vi "Set Control Visibility.vi"(9 "Visible":bool, 10 "index":i32, 11 "Waveform":refnum<vi>) -> ()   [LabVIEW 2016, in "M1M3SupportEUI_Views.lvlib"]
uses:
  M1M3SupportEUI_Views.lvlib
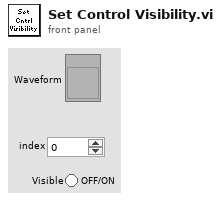
[diagram p1: front panel]
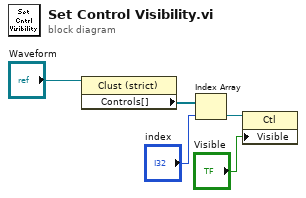
[diagram p0: block diagram]
diagram:
  n1 = property class="Clust (strict)"(reference="Waveform") -> ("Controls[]"=w4:refnum<vi>[])  [unwired: 1 in, 2 out]
  n2 = Index Array(array=w4, index="index") -> (element=w5:refnum<vi>)
  n3 = property class="Ctl"(reference=w5, "Visible"="Visible") -> ()  [unwired: 1 in, 2 out]
